vi "Read (Scaled and Reduced Resolution).vi"(0 "VISA resource name":refnum<visa-resource-name>, 1 "Segment Index (0)":i32 format="%.0g", 5 "Measurement Source (1: Channel 1)":i32(ring)=1 items=["Channel 1"=1, "Channel 2"=2, "Channel 3"=3, "Channel 4"=4, "Function 1"=5, "Function 2"=6, "Function 3"=7, "Function 4"=8, "Memory 1"=9, "Memory 2"=10, "Memory 3"=11, "Memory 4"=12], 7 "Waveform Size (100)":i32=1000 caption="Waveform Size (1000)", 9 "Maximum Time (10000ms)":u32=10000, 11 "error in (no error)":errorcluster) -> (4 "VISA resource name out":refnum<visa-resource-name>, 6 "Waveform Information":T1, 8 "Waveform Data":waveform(dbl)(graph), 15 "error out":errorcluster)   [LabVIEW 2020, in "Agilent 90000 Series.lvlib"]
doc: "Returns a decimated and scaled waveform. If the instrument can perform the decimation before pass it to desktop, a decimated waveform will be read directly from the instrument and returned. Else all waveform points will be read from instrument in chunks and a decimation will be perform in the memory of desktop PC. This VI adopts Min/Max decimating method."
uses:
  Agilent 90000 Series.lvlib
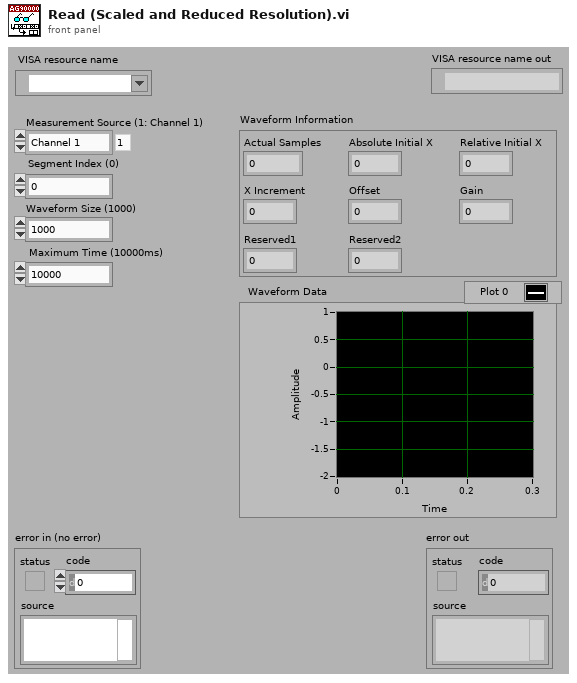
[diagram p1: front panel]
types:
  T1 = cluster{"Actual Samples":i32, "Absolute Initial X":dbl, "Relative Initial X":dbl, "X Increment":dbl, "Offset":dbl, "Gain":dbl, "Reserved1":dbl, "Reserved2":dbl}
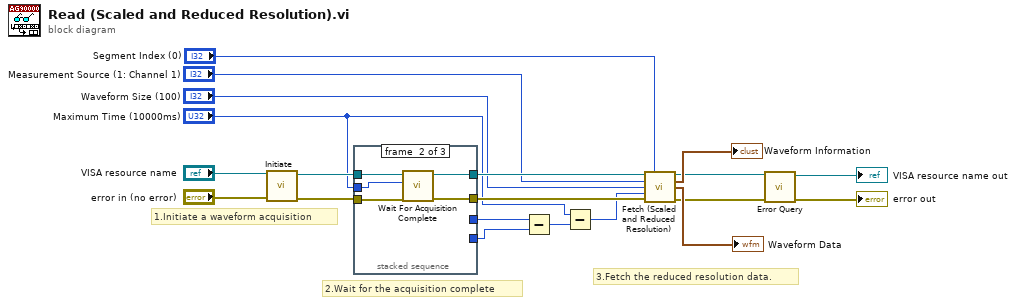
[diagram p0: block diagram]
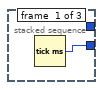
[diagram p2: hidden frame]
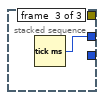
[diagram p3: hidden frame]
diagram:
  # "3.Fetch the reduced resolution data."
  # "2.Wait for the acquisition complete"
  # "1.Initiate a waveform acquisition"
  n1 = call "Initiate.vi"("error in (no error)"="error in (no error)", "VISA resource name"="VISA resource name") -> ("error out"=w17:errorcluster, "VISA resource name out"=w18:refnum<visa-resource-name>)  [unwired: 8 out]
  n2 = stacked-sequence {
    tunnel: [w21 _ _] -> w14
    tunnel: [_ _ w27] -> w15
    tunnel: w18 -> [_ w23 _]
    tunnel: [_ w26 _] -> w13
    tunnel: w17 -> [_ w24 _]
    tunnel: [_ w25 _] -> w12
    tunnel: "Maximum Time (10000ms)" -> [_ w22 _]
    frame #0 {
      n3 = Tick Count (ms)() -> (millisecond timer value=w21:u32)
    }
    frame #1 {
      n4 = call "Wait For Acquisition Complete.vi"("error in (no error)"=w24, "Maximum Time (10000ms)"=w22, "VISA resource name"=w23) -> ("error out"=w25:errorcluster, "VISA resource name out"=w26:refnum<visa-resource-name>)  [unwired: 7 out]
    }
    frame #2 {
      n5 = Tick Count (ms)() -> (millisecond timer value=w27:u32)
    }
  }
  n6 = Subtract(x=w15, y=w14) -> (x-y=w16:u32)
  n7 = Subtract(x="Maximum Time (10000ms)", y=w16) -> (x-y=w9:u32)
  n8 = call "Fetch (Scaled and Reduced Resolution).vi"("VISA resource name"=w13, "Segment Index (0)"="Segment Index (0)", "Measurement Source (1: Channel 1)"="Measurement Source (1: Channel 1)", "Waveform Size (0)"="Waveform Size (100)", "Maximum Time (10000ms)"=w9, "error in (no error)"=w12) -> ("VISA resource name out"=w4:refnum<visa-resource-name>, "Waveform Information"=→"Waveform Information":T1, "Waveform Data"=→"Waveform Data":waveform(dbl), "error out"=w3:errorcluster)  [unwired: 6 out]
  n9 = call "Error Query.vi"("error in (no error)"=w3, "VISA resource name"=w4) -> ("error out"=→"error out":errorcluster, "VISA resource name out"=→"VISA resource name out":refnum<visa-resource-name>)  [unwired: 8 out]
